vi "FindComponentActor.vi"(10 "ActorAlias":string, 11 "Actor":refnum<class "Actor.lvclass">) -> (2 "ComponentActor":T1, 3 "Found":bool)   [LabVIEW 2020, in "jettl.lvlib"]
uses:
  jettl.lvlib
  Actor/Actor.lvclass
  Message/Message.lvclass
  MessageSet.ctl
  Messages.ctl
  Message.ctl
  Actor.ctl
  ActorType.ctl
  TellComponentMap.ctl
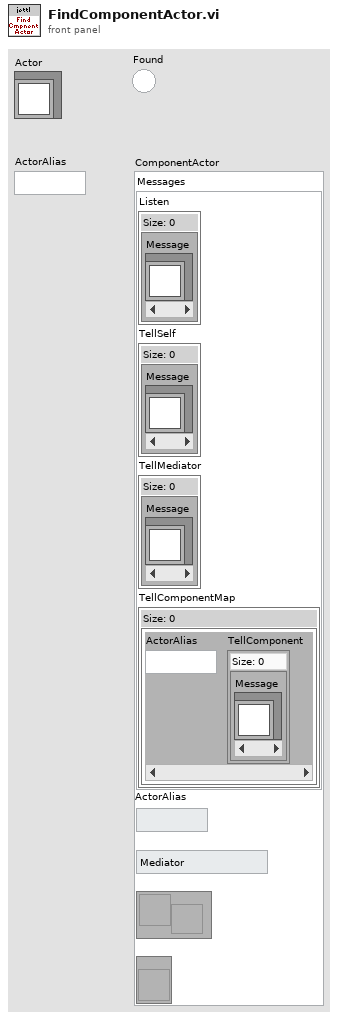
[diagram p1: front panel]
types:
  T1 = typedef "jettl.lvlib/Actor.ctl" = cluster{"Messages":T2, "ActorAlias":string, "ActorType":T5, "Transport":refnum<user-event>, "VIRef":refnum<vi>}
  T2 = typedef "jettl.lvlib/Messages.ctl" = cluster{"Listen":T3, "TellSelf":T3, "TellMediator":T3, "TellComponentMap":T4}
  T3 = typedef "jettl.lvlib/MessageSet.ctl" = set{refnum<class "Message.lvclass">}
  T4 = typedef "jettl.lvlib/TellComponentMap.ctl" = map{string, T3}
  T5 = typedef "jettl.lvlib/ActorType.ctl" = enum16{"Mediator", "Component"}
  T6 = typedef "jettl.lvlib/BaseActor.ctl" = cluster{"Lifetime":T7, "SelfActor":T1, "MediatorActor":T1, "ComponentActorMap":T8}
  T7 = typedef "jettl.lvlib/Lifetime.ctl" = enum16{"Init", "Spawn", "Setup", "TeardownBeforeRunning", "Running", "StopCalled", "StoppingWithComponents", "StoppingNoComponents", "TeardownAfterRunning", "Stopped"}
  T8 = typedef "jettl.lvlib/ComponentActorMap.ctl" = map{string, T1}
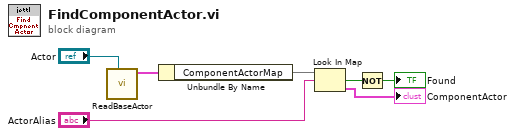
[diagram p0: block diagram]
diagram:
  n1 = call-dynamic "ReadBaseActor.vi"("Actor"="Actor") -> ("BaseActor"=w3:T6)  [unwired: 10 in]
  n2 = Unbundle By Name(w3) -> ("ComponentActorMap"=w1:T8)
  n3 = Look In Map(map=w1, key="ActorAlias") -> (key not found?=w5:bool, value=→"ComponentActor":T1)  [unwired: 1 in]
  n4 = Not(x=w5) -> (.not. x?=→"Found":bool)
